vi "ma_GToLinear.vi"(1 "G unit":bool, 2 "G":dbl format="%0.2f") -> (0 "G (linear)":dbl format="%0.4f")   [LabVIEW 2020, in "NI_MAPro.lvlib"]
uses:
  NI_MAPro.lvlib
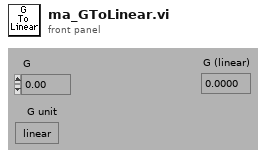
[diagram p1: front panel]
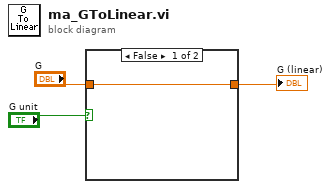
[diagram p0: block diagram]
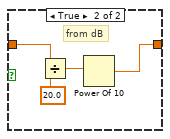
[diagram p2: hidden frame]
diagram:
  n1 = case shown="False" "G unit" {
    tunnel: "G" -> [w4 w7]
    tunnel: [w4 w5] -> w2
    frame False {
    }
    frame True {
      # "from dB"
      n2 = Divide(x=w7, y=20.0) -> (x/y=w6:dbl)
      n3 = Power Of 10(x=w6) -> (10^x=w5:dbl)
    }
  }
  "G (linear)" <- w2
